vi "Decorator3_Example1.vi"() -> ()   [LabVIEW 2020]
uses:
  EncryptedFileDataSource_class/EncryptionType.ctl
  EncryptedFileDataSource_class/EncryptedFileDataSource.lvclass
  FileDataSource_class/FileDataSource.lvclass
panel:
  out "FileContent":string
  out "Return(STRING)":string
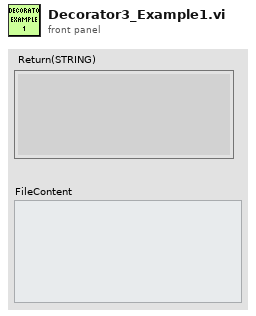
[diagram p1: front panel]
types:
  T1 = typedef "EncryptedFileDataSource.lvclass/EncryptionType.ctl" = enum16{"Type 1", "Type 2"}
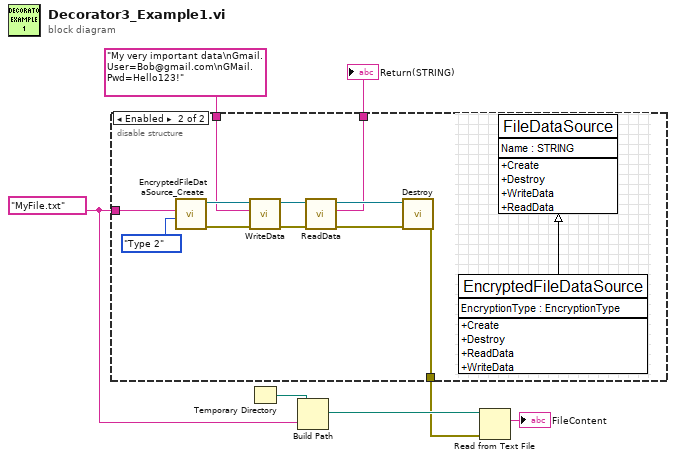
[diagram p0: block diagram]
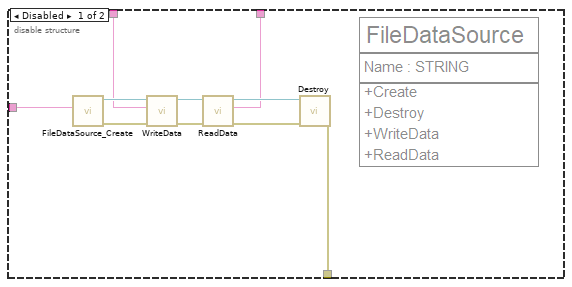
[diagram p2: hidden frame]
diagram:
  w4 = "MyFile.txt" ("Name")
  n1 = disable-structure shown="Enabled" {
    disable-tunnel: "My very important data\nGmail.User=Bob@gmail.com\nGMail.Pwd=Hello123!" ("Data") -> [w11 w22]
    disable-tunnel: [w10 w21] -> w6
    disable-tunnel: w4 -> [w9 w19]
    disable-tunnel: [w8 w20] -> w1
    frame Disabled {
      n2 = call "FileDataSource_Create.vi"("Name"=w9) -> ("error out"=w16:errorcluster, "reference out"=w15:refnum<class "FileDataSource.lvclass">)  [unwired: 9 in]
      n3 = call-dynamic "WriteData.vi"("Error In"=w16, "Data"=w11, "reference in"=w15) -> ("Error Out"=w13:errorcluster, "reference out"=w14:refnum<class "FileDataSource.lvclass">)  [unwired: 7 in]
      n4 = call-dynamic "ReadData.vi"("Error In"=w13, "reference in"=w14) -> ("Error Out"=w12:errorcluster, "Return(STRING)"=w10:string, "reference out"=w17:refnum<class "FileDataSource.lvclass">)  [unwired: 7 in]
      n5 = call-dynamic "Destroy.vi"("error in (no error)"=w12, "reference in"=w17) -> ("error out"=w8:errorcluster)  [unwired: 8 in, 1 out]
    }
    frame Enabled {
      n6 = call "EncryptedFileDataSource_Create.vi"("EncryptionType(Type1)"=EncryptionType."Type 2", "Name"=w19) -> ("error out"=w27:errorcluster, "reference out"=w26:refnum<class "EncryptedFileDataSource.lvclass">)  [unwired: 8 in]
      n7 = call-dynamic "WriteData.vi"("Error In"=w27, "Data"=w22, "reference in"=w26) -> ("Error Out"=w24:errorcluster, "reference in"=w25:refnum<class "EncryptedFileDataSource.lvclass">)  [unwired: 7 in]
      n8 = call-dynamic "ReadData.vi"("Error In"=w24, "reference in"=w25) -> ("Error Out"=w23:errorcluster, "Return(STRING)"=w21:string, "reference in"=w28:refnum<class "EncryptedFileDataSource.lvclass">)  [unwired: 7 in]
      n9 = call-dynamic "Destroy.vi"("error in (no error)"=w23, "reference in"=w28) -> ("error out"=w20:errorcluster)  [unwired: 8 in, 1 out]
    }
  }
  "Return(STRING)" <- w6
  n10 = Temporary Directory() -> (w5:path)
  n11 = Build Path(base path=w5, name or relative path=w4) -> (appended path=w3:path)
  n12 = Read from Text File(file (use dialog)=w3, error in=w1) -> (text=→"FileContent":string)  [unwired: 2 in, 3 out]
